vi "Create Class ObjectData DVR.vi"(8 "error in (no error)":errorcluster, 11 "DLP2 in":refnum<class "DLP2.lvclass">) -> (0 "error out":errorcluster, 3 "DLP2 out":refnum<class "DLP2.lvclass">)   [LabVIEW 2022 SP3, in "DLP2.lvclass"]
doc: "Developed by Kevin Thompson\nkevin@thompsonengineering.net\n\nCopyright 2018\nThompson Engineering, LLC"
uses:
  DLP2.lvclass
  DataTypes/ObjData--cluster.ctl
  DataTypes/Settings--cluster.ctl
  DataTypes/Public Events--cluster.ctl
  Common/Controls/TD Async CmdMsg EventData--cluster.ctl
  Common/Controls/TD Sync API Event Data.ctl
  Common/Controls/APIReturnCluster--Cluster.ctl
  Common/Controls/TD Sync API Task State.ctl
  DataTypes/Dependency--cluster.ctl
  Database/Database.lvclass
  DataTypes/Read Data--cluster.ctl
  DLP2.lvclass/DLP2.ctl
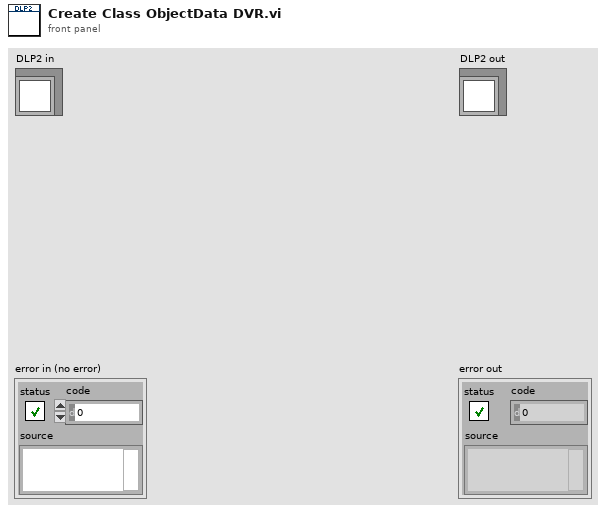
[diagram p1: front panel]
types:
  T1 = typedef "DLP2.lvclass/ObjData--cluster.ctl" = cluster{"Settings":T2, "Public Events":T3, "Dependency":T4, "ReadData-placeholder":T5, "VISA-placeholder":refnum<visa-resource-name>}
  T2 = typedef "DLP2.lvclass/Settings--cluster.ctl" = cluster{"Simulation":bool}
  T3 = typedef "DLP2.lvclass/Public Events--cluster.ctl" = cluster{"Temp01.AsyncCmd Event":refnum<user-event>, "Temp01.AsyncMsg Event":refnum<user-event>, "stop process":refnum<user-event>, "API Incoming Event":refnum<user-event>, "API Executed Event":refnum<user-event>, "API Return Event":refnum<user-event>}
  T4 = typedef "DLP2.lvclass/Dependency--cluster.ctl" = cluster{"Config":refnum<class>, "Database":refnum<class "Database.lvclass">}
  T5 = typedef "DLP2.lvclass/Read Data--cluster.ctl" = cluster{"Data":dbl}
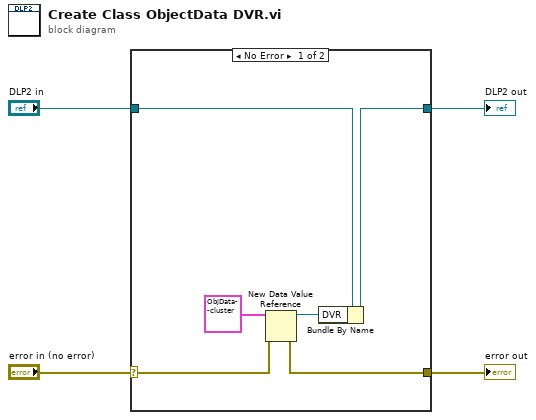
[diagram p0: block diagram]
diagram:
  n1 = case shown="No Error" "error in (no error)" {
    selector: "error in (no error)" -> [w9 w12]
    tunnel: [w8 w12] -> w3
    tunnel: [w6 w11] -> w1
    tunnel: "DLP2 in" -> [w7 w11]
    frame No Error {
      n2 = New Data Value Reference(data value=T1 {"Settings"={"Simulation"=FALSE}, "Public Events"={"Temp01.AsyncCmd Event"=refnum, "Temp01.AsyncMsg Event"=refnum, "stop process"=refnum, "API Incoming Event"=refnum, "API Executed Event"=refnum, "API Return Event"=refnum}, "Dependency"={"Config"=refnum, "Database"=refnum}, "ReadData-placeholder"={"Data"=0.0}, "VISA-placeholder"=""} ("ObjData"), error in=w9) -> (data value reference=w10:refnum<data-value>, error out=w8:errorcluster)
      n3 = Bundle By Name(cluster=w7, "DVR"=w10) -> (w6:refnum<class "DLP2.lvclass">)
    }
    frame Error {
    }
  }
  "error out" <- w3
  "DLP2 out" <- w1
